vi "WPI_MXP General IO to MXP Pin.vi"   [LabVIEW 2017]
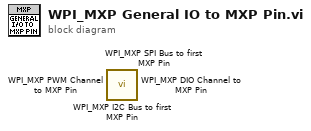
[diagram p0: block diagram]
diagram:
  n1 = call <vilib>:"WPI_MXP I2C Bus to first MXP Pin.vi"() -> ()  [unwired: 15 in, 1 out]
  n2 = call <vilib>:"WPI_MXP SPI Bus to first MXP Pin.vi"() -> ()  [unwired: 15 in, 1 out]
  n3 = call <vilib>:"WPI_MXP PWM Channel to MXP Pin.vi"() -> ()  [unwired: 15 in, 1 out]
  n4 = call <vilib>:"WPI_MXP DIO Channel to MXP Pin.vi"() -> ()  [unwired: 15 in, 1 out]
